vi "main.vi"() -> ()   [LabVIEW 2022 SP3]
uses:
  <vilib>/Instr/_visa.llb/VISA Configure Serial Port (Instr).vi
panel:
  in  "kd2":dbl
  in  "ki2":dbl
  in  "kp2":dbl
  in  "kd1":dbl
  in  "ki1":dbl
  in  "kp1":dbl
  in  "目标ADC":dbl
  out "ENC":u16(graph)
  out "ADC":u16(graph)
  in  "手动起摆":bool
  in  "匀速转动":bool
  in  "起摆":bool
  out "反馈":string
  out "ENC":u16
  out "ADC":u16
  in  "停止":bool
  in  "终止符":u8=10 caption="终止符\n(0xA = '\\n' = LF)" format="%.0x"
  in  "数据比特":u16(ring)=10 caption="停止位（10: 1位）" items=["1.0"=10, "1.5"=15, "2.0"=20]
  in  "data bits (8)":u16=8 caption="数据比特(8)" min=5 max=8 step=1
  in  "启用终止符":bool=TRUE caption="启用终止符 (T)"
  in  "奇偶":enum16{"None", "Odd", "Even", "Mark", "Space"}(ring) caption="奇偶（0:无）"
  in  "baud rate (9600)":u32=9600 caption="波特率(9600)"
  in  "端口":refnum<visa-resource-name> caption="VISA资源名称"
  # "仪表盘"
  # "串口调试"
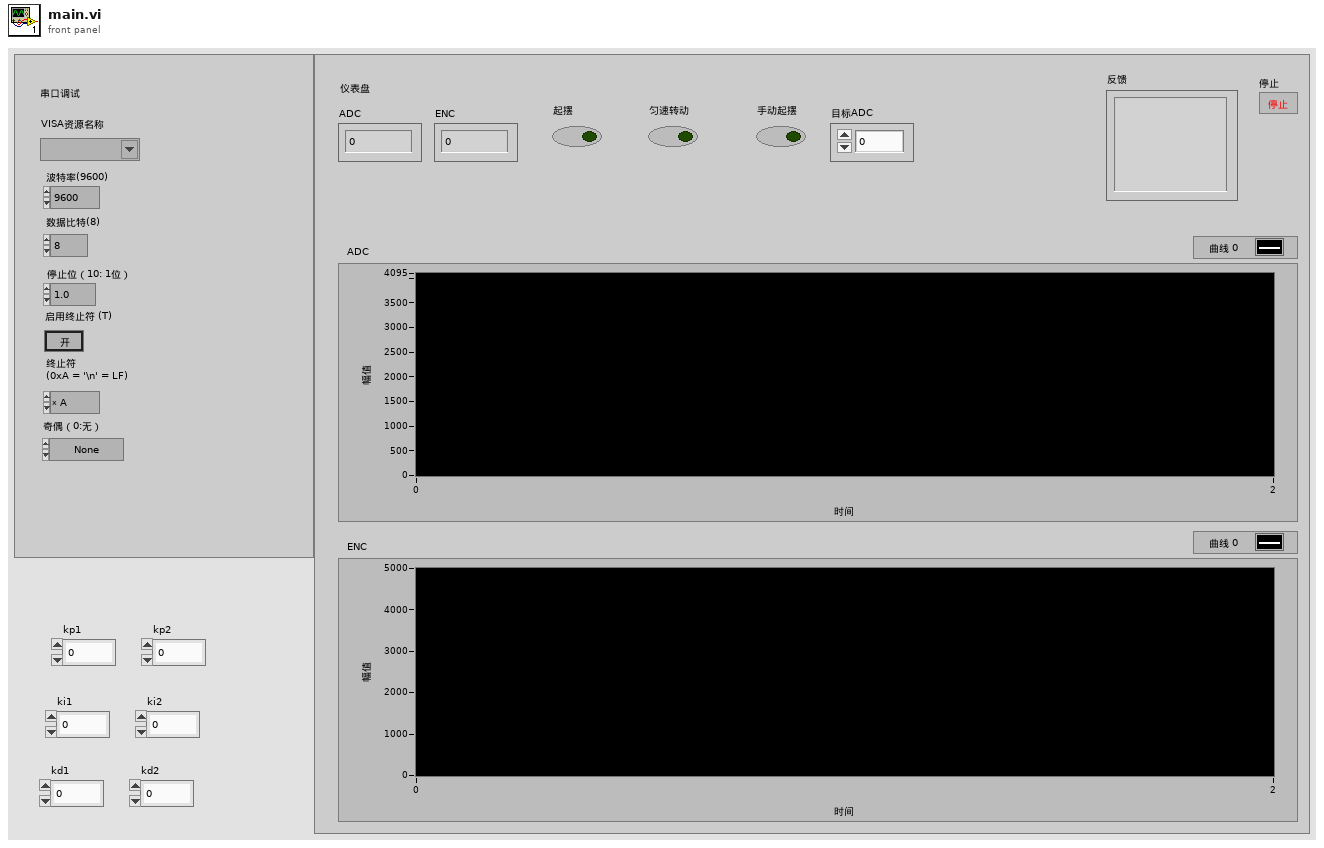
[diagram p1: front panel]
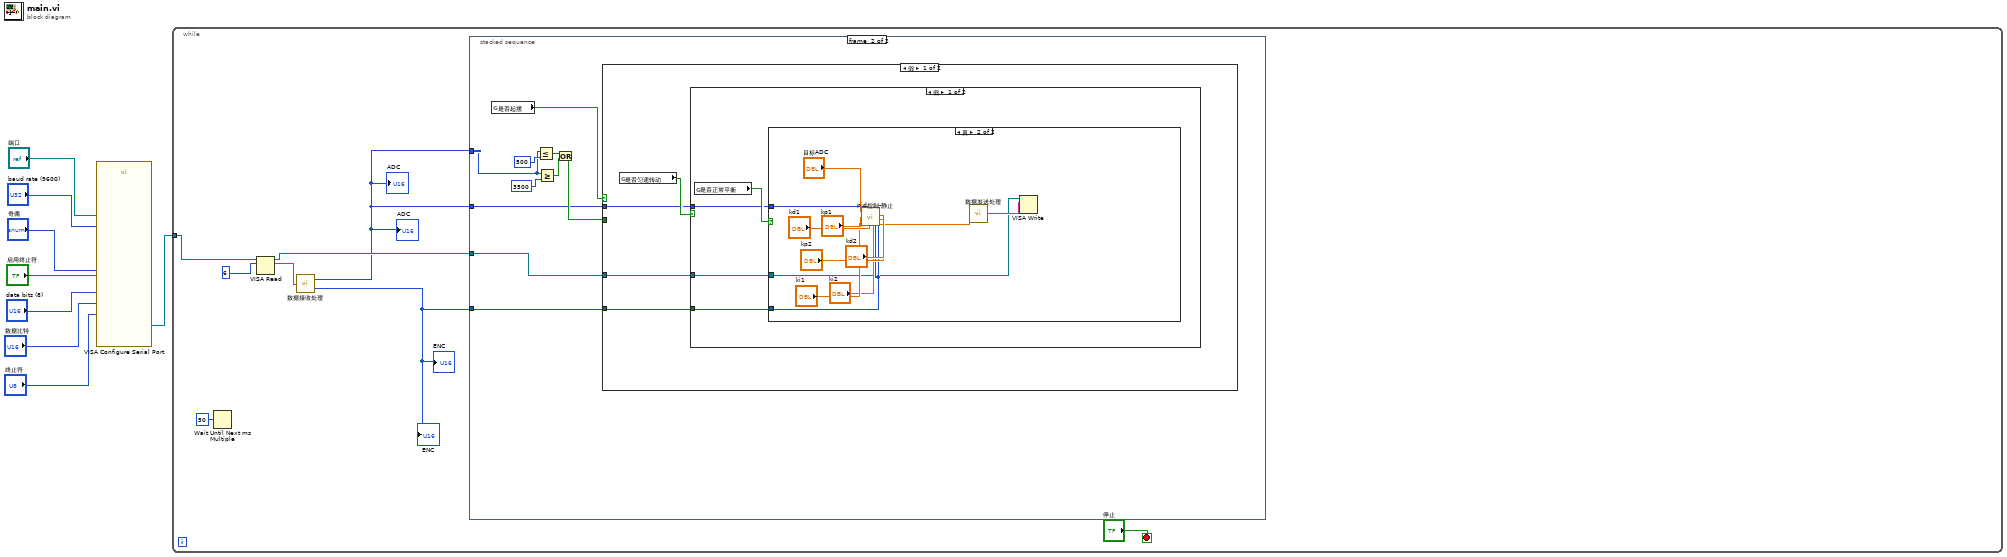
[diagram p0: block diagram]
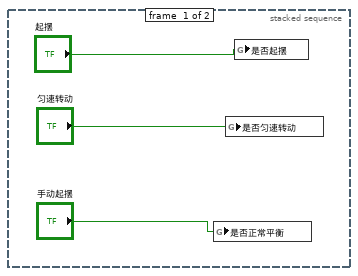
[diagram p2: hidden frame]
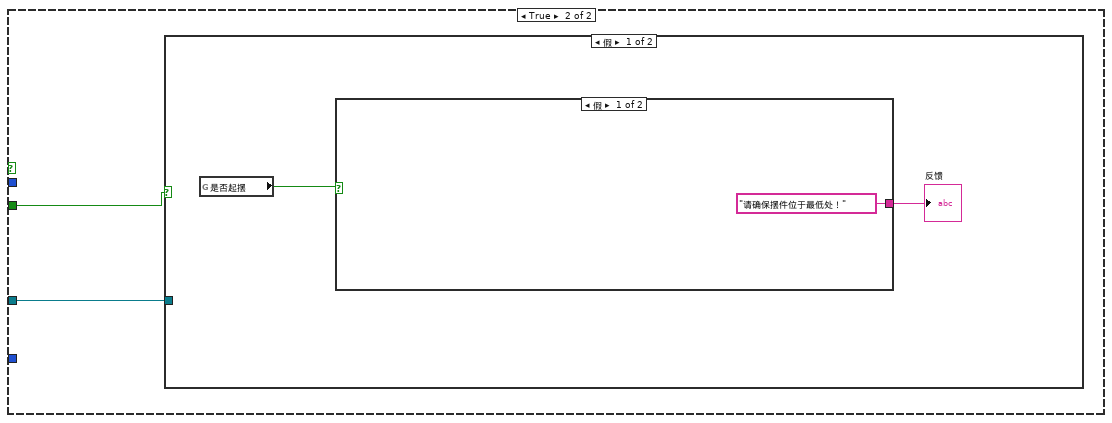
[diagram p5: hidden frame]
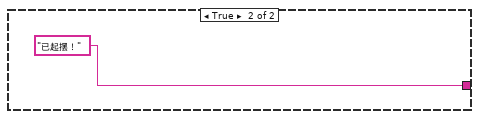
[diagram p6: hidden frame]
diagram:
  n1 = call-poly "VISA Configure Serial Port"("VISA resource name"="端口", "termination char\n(0xA = '\\n' = LF)"="终止符", "Enable Termination\nChar (T)"="启用终止符", "baud rate (9600)"="baud rate (9600)", "data bits (8)"="data bits (8)", "parity (0:none)"="奇偶", "stop bits (10: 1 bit)"="数据比特") -> ("VISA resource name out"=w1:refnum<visa-resource-name>)  [unwired: 7 in, 1 out]
  n2 = while {
    tunnel: w1 -> [w14]
    stop <- "停止" stop-if-true
    n3 = Wait Until Next ms Multiple(millisecond multiple=u32 50 ("毫秒倍数")) -> ()  [unwired: 1 out]
    n4 = VISA Read(VISA resource name=w14, byte count=u32 6 ("字节总数")) -> (VISA resource name out=w12:refnum<visa-resource-name>, read buffer=w11:string)  [unwired: 1 in, 2 out]
    n5 = call "数据接收处理.vi"("字符串"=w11) -> ("ADC"=w10:u16, "ENC"=w9:u16)
    "ADC" <- w10
    "ENC" <- w9
    "ADC" <- w10
    "ENC" <- w9
    n6 = stacked-sequence {
      tunnel: w10 -> [_ w27]
      tunnel: w12 -> [_ w23]
      tunnel: w10 -> [_ w21]
      tunnel: w9 -> [_ w20]
      frame #0 {
        n7 = global write "全局 1.vi" "是否正常平衡"("手动起摆") -> ()
        n8 = global write "全局 1.vi" "是否匀速转动"("匀速转动") -> ()
        n9 = global write "全局 1.vi" "是否起摆"("起摆") -> ()
      }
      frame #1 {
        n10 = global read "全局 1.vi" "是否起摆"() -> (w22:bool)
        n11 = Less Or Equal?(x=w27, y=u16 500) -> (x <= y?=w28:bool)
        n12 = Greater Or Equal?(x=w27, y=u16 3500) -> (x >= y?=w25:bool)
        n13 = Or(x=w28, y=w25) -> (x .or. y?=w24:bool)
        n14 = case shown="假" w22 {
          tunnel: w24 -> [_ w51]
          tunnel: w23 -> [w30 w50]
          tunnel: w21 -> [w32 _]
          tunnel: w20 -> [w31 _]
          frame False {
            n15 = global read "全局 1.vi" "是否匀速转动"() -> (w33:bool)
            n16 = case shown="假" w33 {
              tunnel: w32 -> [w36 _]
              tunnel: w31 -> [w35 _]
              tunnel: w30 -> [w34 _]
              frame False {
                n17 = global read "全局 1.vi" "是否正常平衡"() -> (w37:bool)
                n18 = case shown="真" w37 {
                  tunnel: w36 -> [_ w48]
                  tunnel: w35 -> [_ w41]
                  tunnel: w34 -> [_ w38]
                  frame False {
                  }
                  frame True {
                    n19 = call "pid控制-静止.vi"("目标p1"="目标ADC", "当前p1"=w48, "kp1"="kp1", "ki1"="ki1", "kd1"="kd1", "目标p2"=w41, "当前p2"=w41, "kp2"="kp2", "ki2"="ki2", "kd2"="kd2") -> ("输出v"=w40:dbl)
                    n20 = call "数据发送处理.vi"("PWM"=w40) -> ("字符串"=w39:string)
                    n21 = VISA Write(VISA resource name=w38, write buffer=w39) -> ()  [unwired: 1 in, 3 out]
                  }
                }
              }
              frame True {
              }
            }
          }
          frame True {
            n22 = case shown="假" w51 {
              tunnel: w50 -> [_ _]
              frame False {
                n23 = global read "全局 1.vi" "是否起摆"() -> (w53:bool)
                n24 = case shown="假" w53 {
                  tunnel: ["请确保摆件位于最低处！" ("反馈") "已起摆！" ("反馈")] -> w52
                  frame False {
                  }
                  frame True {
                  }
                }
                "反馈" <- w52
              }
              frame True {
              }
            }
          }
        }
      }
    }
  }
